vi "PulseGeneratorFunction-Single.vi"(2 "Frequency_old (Hz)":dbl, 3 "Ch Setup":T1={"IP Address"="192.168.126.147", "DIO #"=0, "Frequency (Hz)"=200.0, "duty cycle (%)"=0.5, "Enable"=FALSE}, 4 "Mode":T2(ring)) -> (0 "error?":bool)   [LabVIEW 2015]
uses:
  <vilib>/Utility/error.llb/DialogType.ctl
  T7Examples/MODBUS/T7MOD_Write_UINT32_Register.vi
  T7Examples/MODBUS/T7MOD_Write_UINT16_Register.vi
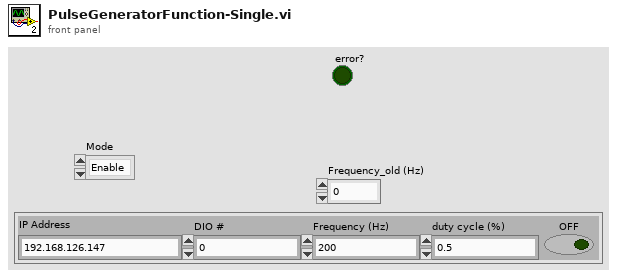
[diagram p1: front panel]
types:
  T1 = cluster{"IP Address":string, "DIO #":u16, "Frequency (Hz)":dbl, "duty cycle (%)":dbl, "Enable":bool}
  T2 = enum16{"Enable", "Disable", "Change Frequency", "Change Duty Cycle", "Configure", "Configure and Run"}
  T3 = typedef "DialogType.ctl" = u16
  T4 = cluster{"Clock Enable":u16, "Divisor":u16, "Roll Value":u16}
  T5 = cluster{"Pulse Enable":u16, "Index":u16, "Duty Cycle":u16}
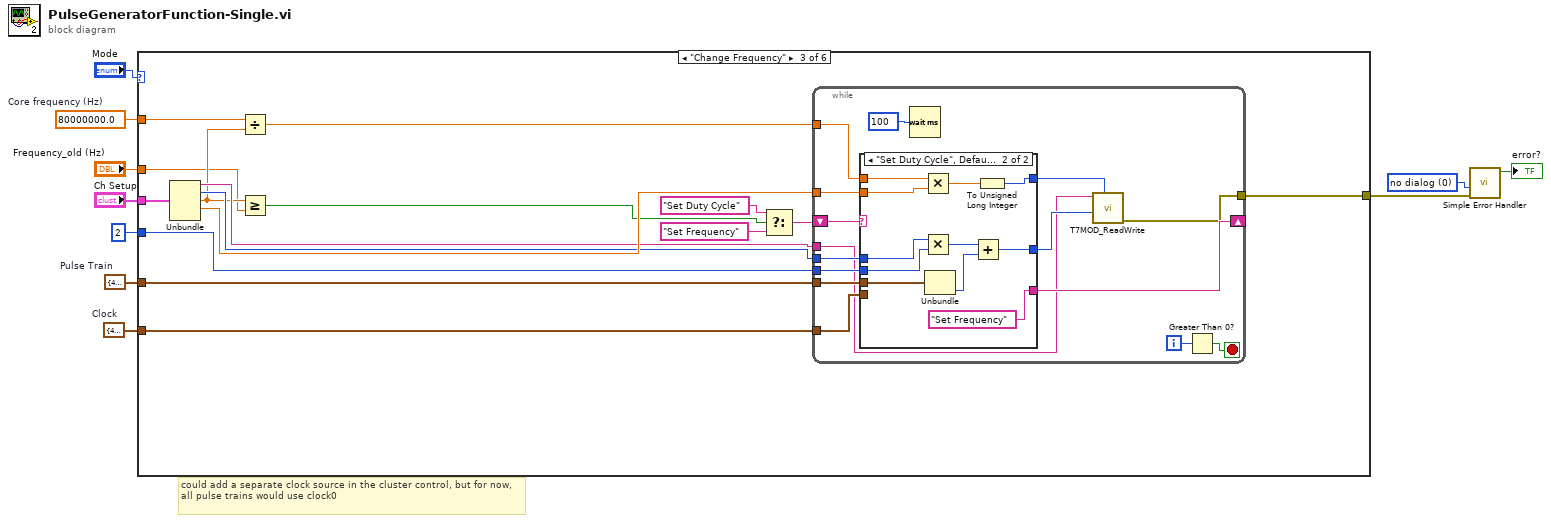
[diagram p0: block diagram]
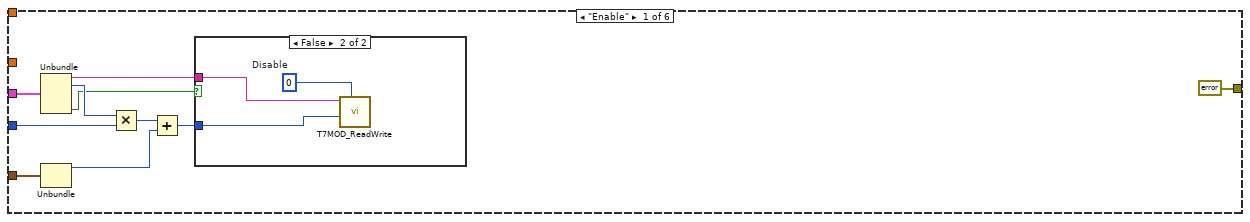
[diagram p2: hidden frame]
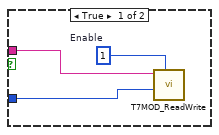
[diagram p3: hidden frame]
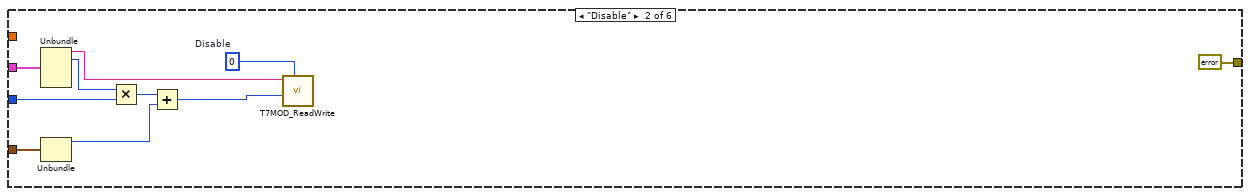
[diagram p4: hidden frame]
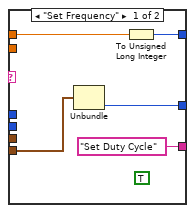
[diagram p5: hidden frame]
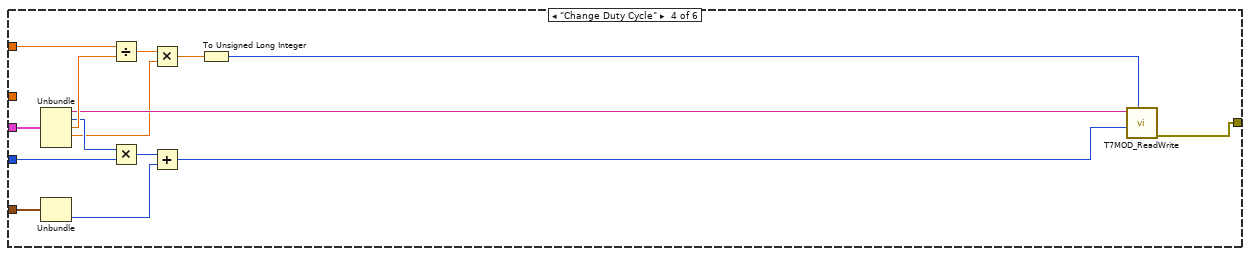
[diagram p6: hidden frame]
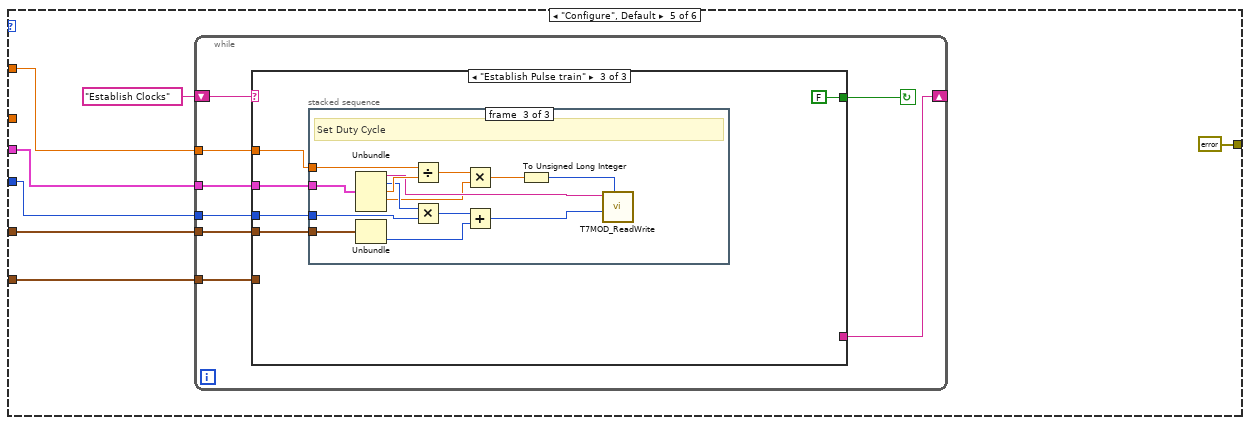
[diagram p7: hidden frame]
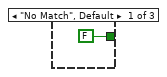
[diagram p8: hidden frame]
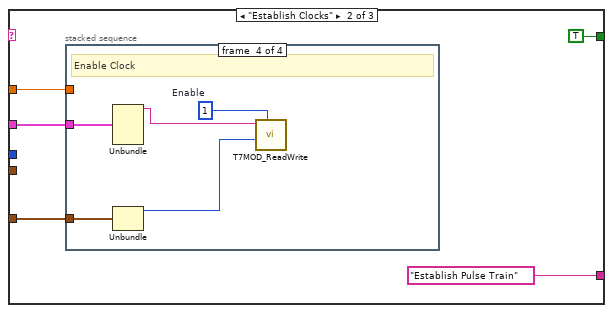
[diagram p9: hidden frame]
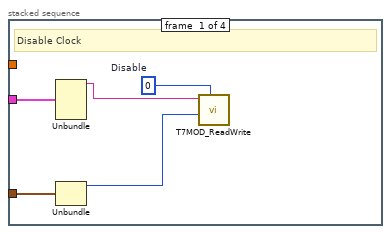
[diagram p10: hidden frame]
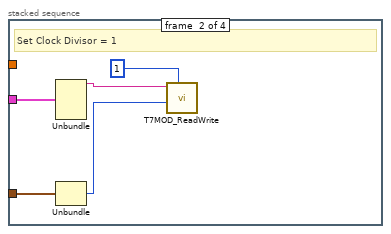
[diagram p11: hidden frame]
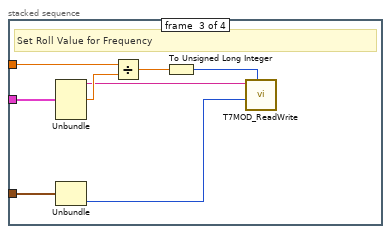
[diagram p12: hidden frame]
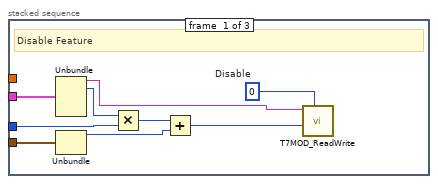
[diagram p13: hidden frame]
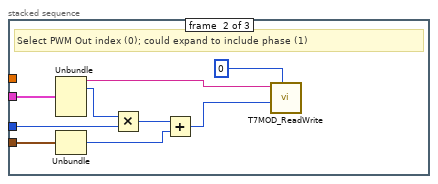
[diagram p14: hidden frame]
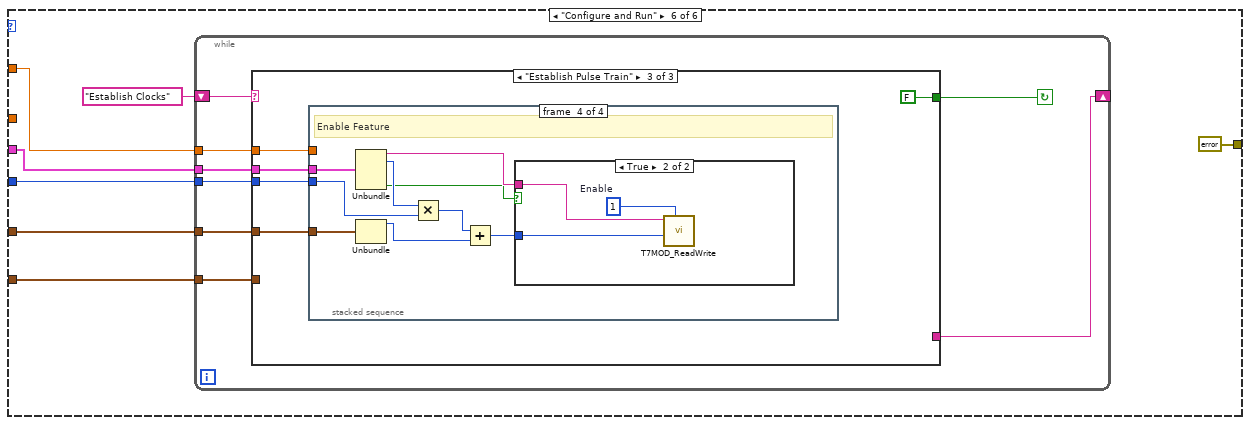
[diagram p15: hidden frame]
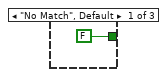
[diagram p16: hidden frame]
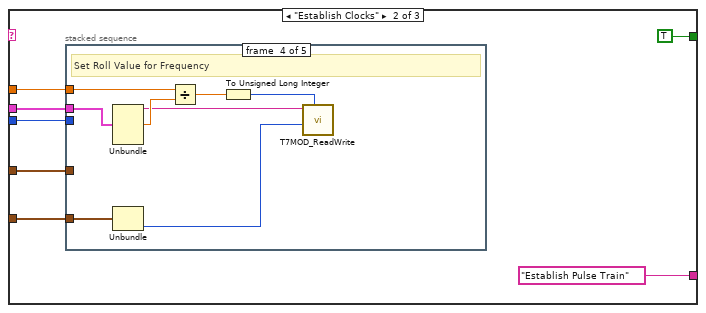
[diagram p17: hidden frame]
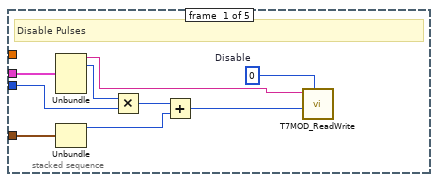
[diagram p18: hidden frame]
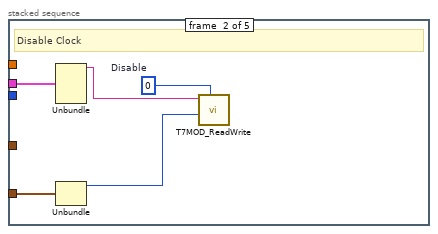
[diagram p19: hidden frame]
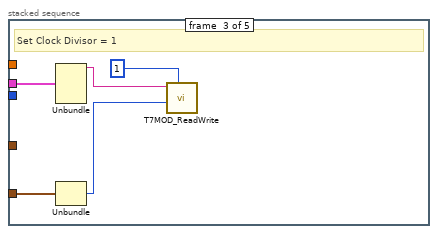
[diagram p20: hidden frame]
diagram:
  w3 = T3 0 items=["no dialog", "OK message", "continue or stop message", "OK message + warnings", "continue/stop + warnings"] ("type of dialog (OK msg:1)")
  w6 = T4 {"Clock Enable"=44900, "Divisor"=44901, "Roll Value"=44904}  # Clock
  w7 = T5 {"Pulse Enable"=44000, "Index"=44100, "Duty Cycle"=44300}  # Pulse Train
  w9 = 80000000.0  # Core frequency (Hz)
  # "could add a separate clock source in the cluster control, but for now, all pulse trains would use clock0"
  n1 = case shown="\"Change Frequency\"" "Mode" {
    tunnel: "Ch Setup" -> [w20 w36 w51 w98 w105 w186]
    tunnel: w9 -> [_ _ w52 w97 w103 w184]
    tunnel: 2 -> [w19 w35 w46 w96 w102 w183]
    tunnel: w7 -> [w18 w34 w50 w95 w101 w182]
    tunnel: w6 -> [_ _ w45 _ w100 w181]
    tunnel: [errorcluster {"status"=FALSE, "code"=0, "source"=""} ("error out") errorcluster {"status"=FALSE, "code"=0, "source"=""} ("error out") w43 w84 errorcluster {"status"=FALSE, "code"=0, "source"=""} ("error out") errorcluster {"status"=FALSE, "code"=0, "source"=""} ("error out")] -> w4
    tunnel: "Frequency_old (Hz)" -> [_ _ w41 _ _ _]
    frame "Enable" {
      n2 = Unbundle(w20) -> ("IP Address"=w13:string, "DIO #"=w17:u16, "Enable"=w12:bool)  [unwired: 2 out]
      n3 = Unbundle(w18) -> ("Pulse Enable"=w15:u16)  [unwired: 2 out]
      n4 = Multiply(x=w17, y=w19) -> (x*y=w16:i32)
      n5 = Add(x=w16, y=w15) -> (x+y=w14:i32)
      n6 = case shown="False" w12 {
        tunnel: w14 -> [w23 w26]
        tunnel: w13 -> [w22 w25]
        frame True {
          w21 = u32 1  # Enable
          n7 = call-poly "T7MOD_ReadWrite.vi"("UINT32 to Write"=w21, "LabJack UINT32 Register"=w23, "Remote IP Address"=w22) -> ()  [unwired: 7 in, 2 out]
        }
        frame False {
          w24 = u32 0  # Disable
          n8 = call-poly "T7MOD_ReadWrite.vi"("UINT32 to Write"=w24, "LabJack UINT32 Register"=w26, "Remote IP Address"=w25) -> ()  [unwired: 7 in, 2 out]
        }
      }
    }
    frame "Disable" {
      w28 = u32 0  # Disable
      n9 = Unbundle(w36) -> ("IP Address"=w29:string, "DIO #"=w33:u16)  [unwired: 3 out]
      n10 = Unbundle(w34) -> ("Pulse Enable"=w31:u16)  [unwired: 2 out]
      n11 = Multiply(x=w33, y=w35) -> (x*y=w32:i32)
      n12 = Add(x=w32, y=w31) -> (x+y=w30:i32)
      n13 = call-poly "T7MOD_ReadWrite.vi"("UINT32 to Write"=w28, "LabJack UINT32 Register"=w30, "Remote IP Address"=w29) -> ()  [unwired: 7 in, 2 out]
    }
    frame "Change Frequency" {
      n14 = Unbundle(w51) -> ("IP Address"=w44:string, "DIO #"=w47:u16, "Frequency (Hz)"=w42:dbl, "duty cycle (%)"=w48:dbl)  [unwired: 1 out]
      n15 = Divide(x=w52, y=w42) -> (x/y=w49:dbl)
      n16 = Greater Or Equal?(x=w42, y=w41) -> (x >= y?=w40:bool)
      n17 = Select(t="Set Duty Cycle", s=w40, f="Set Frequency") -> (s? t:f=w37:string)
      n18 = while {
        shift-right: [w66] -> _
        shift-left: w37 -> [w67]
        tunnel: w50 -> [w63]
        tunnel: w49 -> [w62]
        tunnel: w48 -> [w61]
        tunnel: w47 -> [w60]
        tunnel: w46 -> [w59]
        tunnel: w45 -> [w58]
        tunnel: w44 -> [w57]
        tunnel: [w56] -> w43
        i -> [w54]
        stop <- w53 stop-if-true
        n19 = case shown="\"Set Duty Cycle\", Default" w67 {
          tunnel: ["Set Duty Cycle" "Set Frequency"] -> w66
          tunnel: [w72 w79] -> w65
          tunnel: [w71 w78] -> w64
          tunnel: w63 -> [_ w77]
          tunnel: w62 -> [w69 w76]
          tunnel: w61 -> [_ w75]
          tunnel: w60 -> [_ w74]
          tunnel: w59 -> [_ w73]
          tunnel: w58 -> [w70 _]
          frame "Set Frequency" {
            (unwired) TRUE
            n20 = Unbundle(w70) -> ("Roll Value"=w71:u16)  [unwired: 2 out]
            n21 = To Unsigned Long Integer(number=w69) -> (unsigned 32bit integer=w72:u32)
          }
          frame "Set Duty Cycle", Default {
            n22 = Multiply(x=w76, y=w75) -> (x*y=w82:dbl)
            n23 = Multiply(x=w74, y=w73) -> (x*y=w80:i32)
            n24 = Unbundle(w77) -> ("Duty Cycle"=w81:u16)  [unwired: 2 out]
            n25 = Add(x=w80, y=w81) -> (x+y=w78:i32)
            n26 = To Unsigned Long Integer(number=w82) -> (unsigned 32bit integer=w79:u32)
          }
        }
        n27 = Wait (ms)(milliseconds to wait=u32 100) -> ()  [unwired: 1 out]
        n28 = call-poly "T7MOD_ReadWrite.vi"("UINT32 to Write"=w65, "LabJack UINT32 Register"=w64, "Remote IP Address"=w57) -> ("error out"=w56:errorcluster)  [unwired: 7 in, 1 out]
        n29 = Greater Than 0?(x=w54) -> (x > 0?=w53:bool)
      }
    }
    frame "Change Duty Cycle" {
      n30 = Unbundle(w98) -> ("IP Address"=w88:string, "DIO #"=w93:u16, "Frequency (Hz)"=w94:dbl, "duty cycle (%)"=w85:dbl)  [unwired: 1 out]
      n31 = Unbundle(w95) -> ("Duty Cycle"=w91:u16)  [unwired: 2 out]
      n32 = Divide(x=w97, y=w94) -> (x/y=w86:dbl)
      n33 = Multiply(x=w93, y=w96) -> (x*y=w92:i32)
      n34 = Multiply(x=w86, y=w85) -> (x*y=w87:dbl)
      n35 = Add(x=w92, y=w91) -> (x+y=w89:i32)
      n36 = To Unsigned Long Integer(number=w87) -> (unsigned 32bit integer=w90:u32)
      n37 = call-poly "T7MOD_ReadWrite.vi"("UINT32 to Write"=w90, "LabJack UINT32 Register"=w89, "Remote IP Address"=w88) -> ("error out"=w84:errorcluster)  [unwired: 7 in, 1 out]
    }
    frame "Configure", Default {
      n38 = while {
        tunnel: w103 -> [w112]
        tunnel: w100 -> [w111]
        tunnel: w105 -> [w110]
        tunnel: w101 -> [w109]
        tunnel: w102 -> [w108]
        shift-right: [w107] -> _
        shift-left: "Establish Clocks" -> [w113]
        stop <- w106 continue-if-true
        n39 = case shown="\"Establish Pulse train\"" w113 {
          tunnel: w110 -> [_ w119 w147]
          tunnel: w112 -> [_ w118 w146]
          tunnel: w111 -> [_ w117 _]
          tunnel: w109 -> [_ _ w145]
          tunnel: w108 -> [_ _ w144]
          tunnel: [_ "Establish Pulse Train" _] -> w107
          tunnel: [FALSE TRUE FALSE] -> w106
          frame "No Match", Default {
          }
          frame "Establish Clocks" {
            n40 = stacked-sequence {
              tunnel: w119 -> [w120 w125 w130 w138]
              tunnel: w118 -> [_ _ w137 _]
              tunnel: w117 -> [w124 w129 w136 w142]
              frame #0 {
                w121 = u16 0  # Disable
                # "Disable Clock"
                n41 = Unbundle(w120) -> ("IP Address"=w122:string)  [unwired: 4 out]
                n42 = Unbundle(w124) -> ("Clock Enable"=w123:u16)  [unwired: 2 out]
                n43 = call-poly "T7MOD_ReadWrite.vi"("UINT16 to Write"=w121, "LabJack UINT16 Register"=w123, "Remote IP Address"=w122) -> ()  [unwired: 7 in, 2 out]
              }
              frame #1 {
                # "Set Clock Divisor = 1"
                n44 = Unbundle(w125) -> ("IP Address"=w128:string)  [unwired: 4 out]
                n45 = Unbundle(w129) -> ("Divisor"=w126:u16)  [unwired: 2 out]
                n46 = call-poly "T7MOD_ReadWrite.vi"("UINT16 to Write"=u16 1 ("Disable"), "LabJack UINT16 Register"=w126, "Remote IP Address"=w128) -> ()  [unwired: 7 in, 2 out]
              }
              frame #2 {
                # "Set Roll Value for Frequency"
                n47 = Unbundle(w130) -> ("IP Address"=w131:string, "Frequency (Hz)"=w135:dbl)  [unwired: 3 out]
                n48 = Unbundle(w136) -> ("Roll Value"=w133:u16)  [unwired: 2 out]
                n49 = Divide(x=w137, y=w135) -> (x/y=w134:dbl)
                n50 = To Unsigned Long Integer(number=w134) -> (unsigned 32bit integer=w132:u32)
                n51 = call-poly "T7MOD_ReadWrite.vi"("UINT32 to Write"=w132, "LabJack UINT32 Register"=w133, "Remote IP Address"=w131) -> ()  [unwired: 7 in, 2 out]
              }
              frame #3 {
                w139 = u16 1  # Enable
                # "Enable Clock"
                n52 = Unbundle(w138) -> ("IP Address"=w140:string)  [unwired: 4 out]
                n53 = Unbundle(w142) -> ("Clock Enable"=w141:u16)  [unwired: 2 out]
                n54 = call-poly "T7MOD_ReadWrite.vi"("UINT16 to Write"=w139, "LabJack UINT16 Register"=w141, "Remote IP Address"=w140) -> ()  [unwired: 7 in, 2 out]
              }
            }
          }
          frame "Establish Pulse train" {
            n55 = stacked-sequence {
              tunnel: w147 -> [w156 w165 w179]
              tunnel: w146 -> [_ _ w178]
              tunnel: w145 -> [w155 w164 w177]
              tunnel: w144 -> [w154 w163 w176]
              frame #0 {
                w148 = u32 0  # Disable
                # "Disable Feature"
                n56 = Unbundle(w156) -> ("IP Address"=w149:string, "DIO #"=w153:u16)  [unwired: 3 out]
                n57 = Unbundle(w155) -> ("Pulse Enable"=w151:u16)  [unwired: 2 out]
                n58 = Multiply(x=w153, y=w154) -> (x*y=w152:i32)
                n59 = Add(x=w152, y=w151) -> (x+y=w150:i32)
                n60 = call-poly "T7MOD_ReadWrite.vi"("UINT32 to Write"=w148, "LabJack UINT32 Register"=w150, "Remote IP Address"=w149) -> ()  [unwired: 7 in, 2 out]
              }
              frame #1 {
                # "Select PWM Out index (0); could expand to include phase (1)"
                n61 = Unbundle(w165) -> ("IP Address"=w159:string, "DIO #"=w162:u16)  [unwired: 3 out]
                n62 = Unbundle(w164) -> ("Index"=w157:u16)  [unwired: 2 out]
                n63 = Multiply(x=w162, y=w163) -> (x*y=w161:i32)
                n64 = Add(x=w161, y=w157) -> (x+y=w160:i32)
                n65 = call-poly "T7MOD_ReadWrite.vi"("UINT32 to Write"=u32 0 ("Disable"), "LabJack UINT32 Register"=w160, "Remote IP Address"=w159) -> ()  [unwired: 7 in, 2 out]
              }
              frame #2 {
                # "Set Duty Cycle"
                n66 = Unbundle(w179) -> ("IP Address"=w169:string, "DIO #"=w174:u16, "Frequency (Hz)"=w175:dbl, "duty cycle (%)"=w166:dbl)  [unwired: 1 out]
                n67 = Unbundle(w177) -> ("Duty Cycle"=w172:u16)  [unwired: 2 out]
                n68 = Divide(x=w178, y=w175) -> (x/y=w167:dbl)
                n69 = Multiply(x=w174, y=w176) -> (x*y=w173:i32)
                n70 = Multiply(x=w167, y=w166) -> (x*y=w168:dbl)
                n71 = Add(x=w173, y=w172) -> (x+y=w170:i32)
                n72 = To Unsigned Long Integer(number=w168) -> (unsigned 32bit integer=w171:u32)
                n73 = call-poly "T7MOD_ReadWrite.vi"("UINT32 to Write"=w171, "LabJack UINT32 Register"=w170, "Remote IP Address"=w169) -> ()  [unwired: 7 in, 2 out]
              }
            }
          }
        }
      }
    }
    frame "Configure and Run" {
      n74 = while {
        tunnel: w184 -> [w193]
        tunnel: w181 -> [w192]
        tunnel: w186 -> [w191]
        tunnel: w182 -> [w190]
        tunnel: w183 -> [w189]
        shift-right: [w188] -> _
        shift-left: "Establish Clocks" -> [w194]
        stop <- w187 continue-if-true
        n75 = case shown="\"Establish Pulse Train\"" w194 {
          tunnel: w191 -> [_ w202 w239]
          tunnel: w193 -> [_ w201 w238]
          tunnel: w192 -> [_ w200 _]
          tunnel: w190 -> [_ w197 w237]
          tunnel: w189 -> [_ w196 w236]
          tunnel: [_ "Establish Pulse Train" _] -> w188
          tunnel: [FALSE TRUE FALSE] -> w187
          frame "No Match", Default {
          }
          frame "Establish Clocks" {
            n76 = stacked-sequence {
              tunnel: w202 -> [w211 w212 w217 w222 w230]
              tunnel: w201 -> [_ _ _ w229 _]
              tunnel: w200 -> [_ w216 w221 w228 w234]
              tunnel: w197 -> [w210 _ _ _ _]
              tunnel: w196 -> [w209 _ _ _ _]
              frame #0 {
                w203 = u32 0  # Disable
                # "Disable Pulses"
                n77 = Unbundle(w211) -> ("IP Address"=w204:string, "DIO #"=w208:u16)  [unwired: 3 out]
                n78 = Unbundle(w210) -> ("Pulse Enable"=w206:u16)  [unwired: 2 out]
                n79 = Multiply(x=w208, y=w209) -> (x*y=w207:i32)
                n80 = Add(x=w207, y=w206) -> (x+y=w205:i32)
                n81 = call-poly "T7MOD_ReadWrite.vi"("UINT32 to Write"=w203, "LabJack UINT32 Register"=w205, "Remote IP Address"=w204) -> ()  [unwired: 7 in, 2 out]
              }
              frame #1 {
                w213 = u16 0  # Disable
                # "Disable Clock"
                n82 = Unbundle(w212) -> ("IP Address"=w214:string)  [unwired: 4 out]
                n83 = Unbundle(w216) -> ("Clock Enable"=w215:u16)  [unwired: 2 out]
                n84 = call-poly "T7MOD_ReadWrite.vi"("UINT16 to Write"=w213, "LabJack UINT16 Register"=w215, "Remote IP Address"=w214) -> ()  [unwired: 7 in, 2 out]
              }
              frame #2 {
                # "Set Clock Divisor = 1"
                n85 = Unbundle(w217) -> ("IP Address"=w220:string)  [unwired: 4 out]
                n86 = Unbundle(w221) -> ("Divisor"=w218:u16)  [unwired: 2 out]
                n87 = call-poly "T7MOD_ReadWrite.vi"("UINT16 to Write"=u16 1 ("Disable"), "LabJack UINT16 Register"=w218, "Remote IP Address"=w220) -> ()  [unwired: 7 in, 2 out]
              }
              frame #3 {
                # "Set Roll Value for Frequency"
                n88 = Unbundle(w222) -> ("IP Address"=w223:string, "Frequency (Hz)"=w227:dbl)  [unwired: 3 out]
                n89 = Unbundle(w228) -> ("Roll Value"=w225:u16)  [unwired: 2 out]
                n90 = Divide(x=w229, y=w227) -> (x/y=w226:dbl)
                n91 = To Unsigned Long Integer(number=w226) -> (unsigned 32bit integer=w224:u32)
                n92 = call-poly "T7MOD_ReadWrite.vi"("UINT32 to Write"=w224, "LabJack UINT32 Register"=w225, "Remote IP Address"=w223) -> ()  [unwired: 7 in, 2 out]
              }
              frame #4 {
                w231 = u16 1  # Enable
                # "Enable Clock"
                n93 = Unbundle(w230) -> ("IP Address"=w232:string)  [unwired: 4 out]
                n94 = Unbundle(w234) -> ("Clock Enable"=w233:u16)  [unwired: 2 out]
                n95 = call-poly "T7MOD_ReadWrite.vi"("UINT16 to Write"=w231, "LabJack UINT16 Register"=w233, "Remote IP Address"=w232) -> ()  [unwired: 7 in, 2 out]
              }
            }
          }
          frame "Establish Pulse Train" {
            n96 = stacked-sequence {
              tunnel: w239 -> [w248 w257 w271 w280]
              tunnel: w238 -> [_ _ w270 _]
              tunnel: w237 -> [w247 w256 w269 w279]
              tunnel: w236 -> [w246 w255 w268 w278]
              frame #0 {
                w240 = u32 0  # Disable
                # "Disable Feature"
                n97 = Unbundle(w248) -> ("IP Address"=w241:string, "DIO #"=w245:u16)  [unwired: 3 out]
                n98 = Unbundle(w247) -> ("Pulse Enable"=w243:u16)  [unwired: 2 out]
                n99 = Multiply(x=w245, y=w246) -> (x*y=w244:i32)
                n100 = Add(x=w244, y=w243) -> (x+y=w242:i32)
                n101 = call-poly "T7MOD_ReadWrite.vi"("UINT32 to Write"=w240, "LabJack UINT32 Register"=w242, "Remote IP Address"=w241) -> ()  [unwired: 7 in, 2 out]
              }
              frame #1 {
                # "Select PWM Out index (0); could expand to include phase (1)"
                n102 = Unbundle(w257) -> ("IP Address"=w251:string, "DIO #"=w254:u16)  [unwired: 3 out]
                n103 = Unbundle(w256) -> ("Index"=w249:u16)  [unwired: 2 out]
                n104 = Multiply(x=w254, y=w255) -> (x*y=w253:i32)
                n105 = Add(x=w253, y=w249) -> (x+y=w252:i32)
                n106 = call-poly "T7MOD_ReadWrite.vi"("UINT32 to Write"=u32 0 ("Disable"), "LabJack UINT32 Register"=w252, "Remote IP Address"=w251) -> ()  [unwired: 7 in, 2 out]
              }
              frame #2 {
                # "Set Duty Cycle"
                n107 = Unbundle(w271) -> ("IP Address"=w261:string, "DIO #"=w266:u16, "Frequency (Hz)"=w267:dbl, "duty cycle (%)"=w258:dbl)  [unwired: 1 out]
                n108 = Unbundle(w269) -> ("Duty Cycle"=w264:u16)  [unwired: 2 out]
                n109 = Divide(x=w270, y=w267) -> (x/y=w259:dbl)
                n110 = Multiply(x=w266, y=w268) -> (x*y=w265:i32)
                n111 = Multiply(x=w259, y=w258) -> (x*y=w260:dbl)
                n112 = Add(x=w265, y=w264) -> (x+y=w262:i32)
                n113 = To Unsigned Long Integer(number=w260) -> (unsigned 32bit integer=w263:u32)
                n114 = call-poly "T7MOD_ReadWrite.vi"("UINT32 to Write"=w263, "LabJack UINT32 Register"=w262, "Remote IP Address"=w261) -> ()  [unwired: 7 in, 2 out]
              }
              frame #3 {
                # "Enable Feature"
                n115 = Unbundle(w280) -> ("IP Address"=w273:string, "DIO #"=w277:u16, "Enable"=w272:bool)  [unwired: 2 out]
                n116 = Unbundle(w279) -> ("Pulse Enable"=w275:u16)  [unwired: 2 out]
                n117 = Multiply(x=w277, y=w278) -> (x*y=w276:i32)
                n118 = Add(x=w276, y=w275) -> (x+y=w274:i32)
                n119 = case shown="True" w272 {
                  tunnel: w274 -> [_ w283]
                  tunnel: w273 -> [_ w282]
                  frame False {
                  }
                  frame True {
                    w281 = u32 1  # Enable
                    n120 = call-poly "T7MOD_ReadWrite.vi"("UINT32 to Write"=w281, "LabJack UINT32 Register"=w283, "Remote IP Address"=w282) -> ()  [unwired: 7 in, 2 out]
                  }
                }
              }
            }
          }
        }
      }
    }
  }
  n121 = call <vilib>:"Simple Error Handler.vi"("type of dialog (OK msg:1)"=w3, "error in (no error)"=w4) -> ("error?"=→"error?":bool)  [unwired: 3 in, 4 out]
